vi "Parse TXT Configuration File_Parse DMA Blocks.vi"(8 "error in (no error)":errorcluster, 11 "Array in":string[][](array[string])) -> (0 "error out":errorcluster, 2 "DMA Blocks":T1[](array[typedef]), 3 "Array Out":string[][](array[string]))   [LabVIEW 2017, in "GE_RM_System Explorer.lvlib"]
uses:
  GE_RM_System Explorer.lvlib
  Typedef_DMA Block Settings.ctl
  Shared/Data Channel Type.ctl
  <userlib>/_OpenG.lib/array/array.llb/Remove Duplicates from 1D Array (String)__ogtk.vi
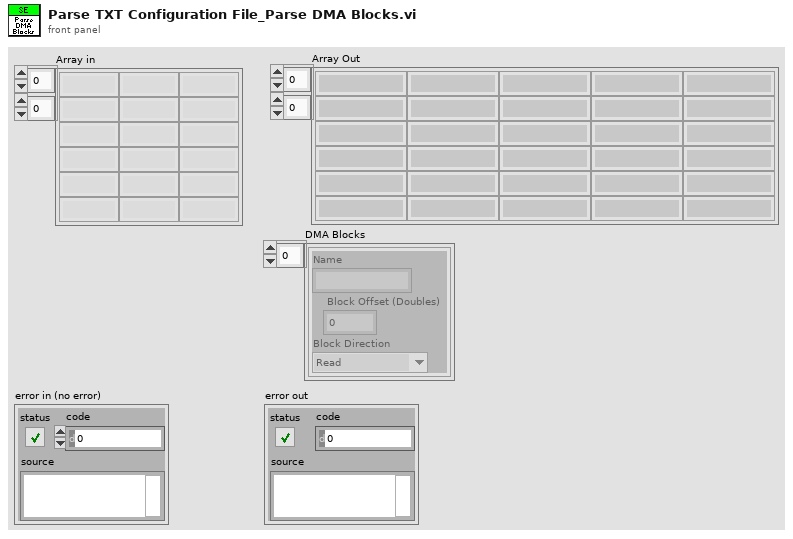
[diagram p1: front panel]
types:
  T1 = typedef "GE_RM_System Explorer.lvlib/Typedef_DMA Block Settings.ctl" = cluster{"Name":string, " Block Offset (Doubles)":u32, "Block Direction":T2}
  T2 = typedef "GE_RM_System Explorer.lvlib/Data Channel Type.ctl" = enum16{"Read", "Write"}
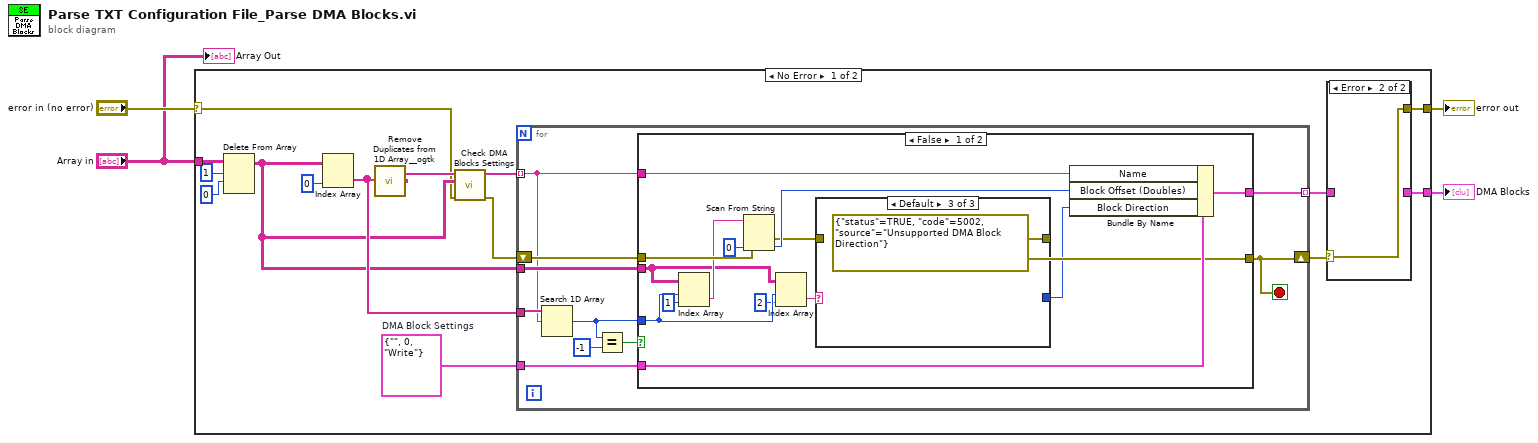
[diagram p0: block diagram]
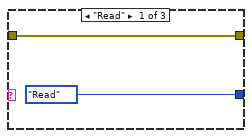
[diagram p3: hidden frame]
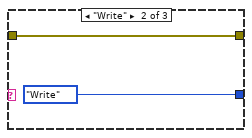
[diagram p4: hidden frame]
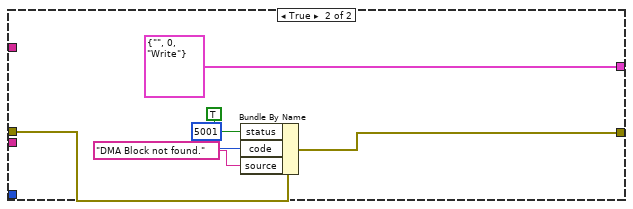
[diagram p5: hidden frame]
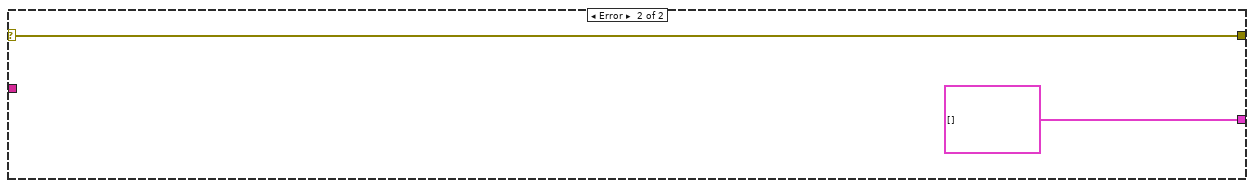
[diagram p6: hidden frame]
diagram:
  n1 = case shown="No Error" "error in (no error)" {
    selector: "error in (no error)" -> [w6 w59]
    tunnel: "Array in" -> [w17 _]
    tunnel: [w11 T1[] []] -> w2
    tunnel: [w10 w59] -> w3
    frame No Error {
      w15 = T1 {"Name"="", " Block Offset (Doubles)"=0, "Block Direction"=enum."Write"}  # DMA Block Settings
      n2 = Delete From Array(array=w17, length=1, index (row)=0) -> (array with subset deleted=w8:string[][])  [unwired: 1 in, 1 out]
      n3 = Index Array(array=w8, index (col)=0 ("disabled index (col)")) -> (element=w14:string[])  [unwired: 1 in]
      n4 = call-poly <userlib>:"Remove Duplicates from 1D Array__ogtk.vi"("Input Array"=w14) -> ("Output Array"=w9:string[])  [unwired: 1 out]
      n5 = call "Check DMA Blocks Settings.vi"("error in (no error)"=w6, "Array in"=w8, "DMA Blocks Names In"=w9) -> ("error out"=w5:errorcluster, "DMA Blocks Names Out"=w7:string[])  [unwired: 7 in]
      n6 = for {
        tunnel: w7 -> [w23] mode=indexing
        tunnel: w15 -> [w32]
        tunnel: [w31] -> w12 mode=indexing
        tunnel: w14 -> [w30]
        tunnel: w8 -> [w26]
        shift-right: [w24] -> w13
        shift-left: w5 -> [w25]
        stop <- w24 stop-if-true
        n7 = Search 1D Array(1D array=w30, element=w23) -> (index of element=w27:i32)  [unwired: 1 in]
        n8 = Equal?(x=w27, y=-1) -> (x = y?=w28:bool)
        n9 = case shown="False" w28 {
          tunnel: w32 -> [w47 _]
          tunnel: [w46 T1 {"Name"="", " Block Offset (Doubles)"=0, "Block Direction"=enum."Write"} ("DMA Block Settings")] -> w31
          tunnel: w23 -> [w45 _]
          tunnel: w27 -> [w38 _]
          tunnel: w26 -> [w39 _]
          tunnel: w25 -> [w43 w57]
          tunnel: [w34 w56] -> w24
          frame False {
            n10 = Index Array(array=w39, index (row)=w38, index (col)=1 ("disabled index (col)")) -> (element=w42:string)
            n11 = Scan From String(input string=w42, error in=w43, default 1=u32 0) -> (error out=w35:errorcluster, output 1=w40:u32)  [unwired: 2 in, 2 out]
            n12 = Index Array(array=w39, index (row)=w38, index (col)=2 ("disabled index (col)")) -> (element=w36:string)
            n13 = case shown="Default" w36 {
              tunnel: w35 -> [w49 w51 _]
              tunnel: [w49 w51 errorcluster {"status"=TRUE, "code"=5002, "source"="Unsupported DMA Block Direction"} ("error IO")] -> w34
              tunnel: [Data_Channel_Type."Read" ("Block Direction") Data_Channel_Type."Write" ("Block Direction") _] -> w33
              frame "Read" {
              }
              frame "Write" {
              }
              frame Default {
              }
            }
            n14 = Bundle By Name(cluster=w47, "Name"=w45, "Block Offset (Doubles)"=w40, "Block Direction"=w33) -> (w46:T1)
          }
          frame True {
            n15 = Bundle By Name(cluster=w57, "status"=TRUE, "code"=5001, "source"="DMA Block not found.") -> (w56:errorcluster)
          }
        }
      }
      n16 = case shown="Error" w13 {
        selector: w13 -> [w20 w22]
        tunnel: w12 -> [w21 _]
        tunnel: [w21 _] -> w11
        tunnel: [w20 w22] -> w10
        frame No Error {
        }
        frame Error {
        }
      }
    }
    frame Error {
    }
  }
  "error out" <- w3
  "DMA Blocks" <- w2
  "Array Out" <- "Array in"
